vi "template.vi"() -> ()   [LabVIEW 2018]
panel:
  out "Arm System":bool
  in  "Start":bool
  out "Laser 2":bool
  out "Laser 1":bool
  in  "Speed Threshold (km/h)":dbl
  out "Safety System 2":bool[](array[boolean])
  out "Safety System 1":bool[](array[boolean])
  out "GPS":cluster{"Lat":dbl, "Lon":dbl, "Speed":dbl}
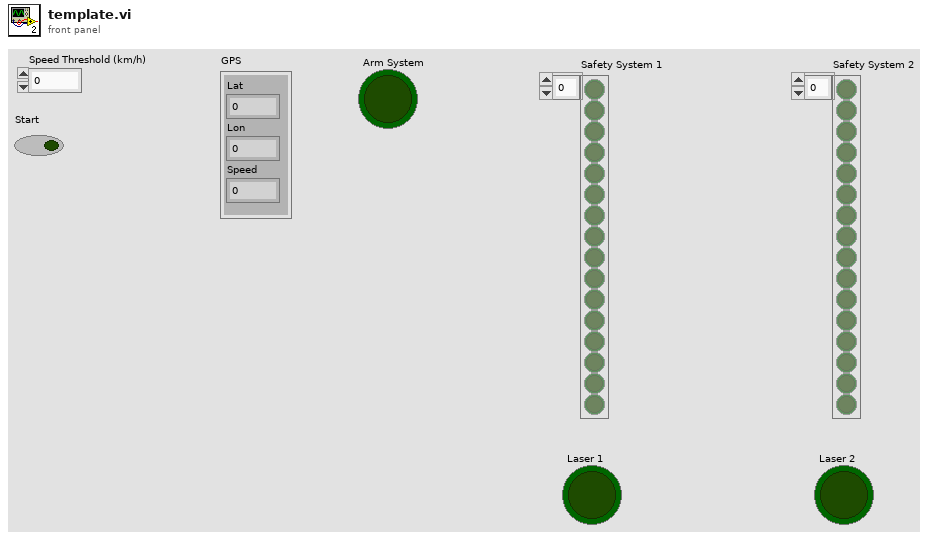
[diagram p1: front panel]
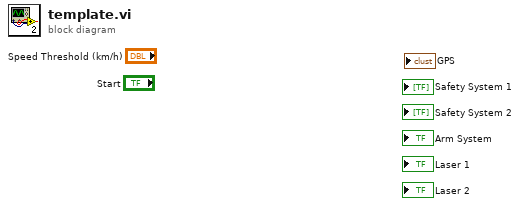
[diagram p0: block diagram]
diagram:
